vi "PGrafica.vi"() -> ()   [LabVIEW 2020]
uses:
  Pos_modifi.vi
  Llenado.vi
  sensores.vi
  Pos_iniciales.vi
  Pos_iniciales3.vi
  Pos_iniciales1.vi
panel:
  out "Piston C":bool
  out "Piston Abierto Y":i32
  out "Piston Abierto X":i32
  out "Sensor 1 Y":i32
  out "Laminadora":bool
  out "Caja Y":i32
  out "Caja X":i32
  out "Caja":bool
  out "Bote Pintado Y":i32
  out "Bote Pintado X":i32
  out "Bote cerrado Y":i32
  out "Bote cerrado X":i32
  out "Carrito Y":i32
  out "Carrito X":i32
  out "Pintura Y":i32
  out "Pintura X":i32
  out "Pintado":dbl(knob) scale=0.0..10.0
  out "Laminadora Y":i32
  out "Laminadora X":i32
  out "Piston cerrado Y":i32
  out "Piston cerrado X":i32
  out "Sensor 1":bool
  out "Bote":u8(slide) scale=0.0..100.0
  out "Mezc Y":i32
  out "Mezc X":i32
  out "Bote Y":i32
  out "Bote X":i32
  out "Sensor1 X":i32
  out "Llenador Y":i32
  out "Llenador X":i32
  out "Llenar":u8(slide) scale=0.0..100.0
  out "Tanque":u8(slide) scale=0.0..100.0
  out "Mezclador":dbl(slide) scale=0.0..10.0
  out "Carrito":bool
  out "Bote Cerrado":bool
  out "Bote Pintado":bool
  out "Piston A":bool
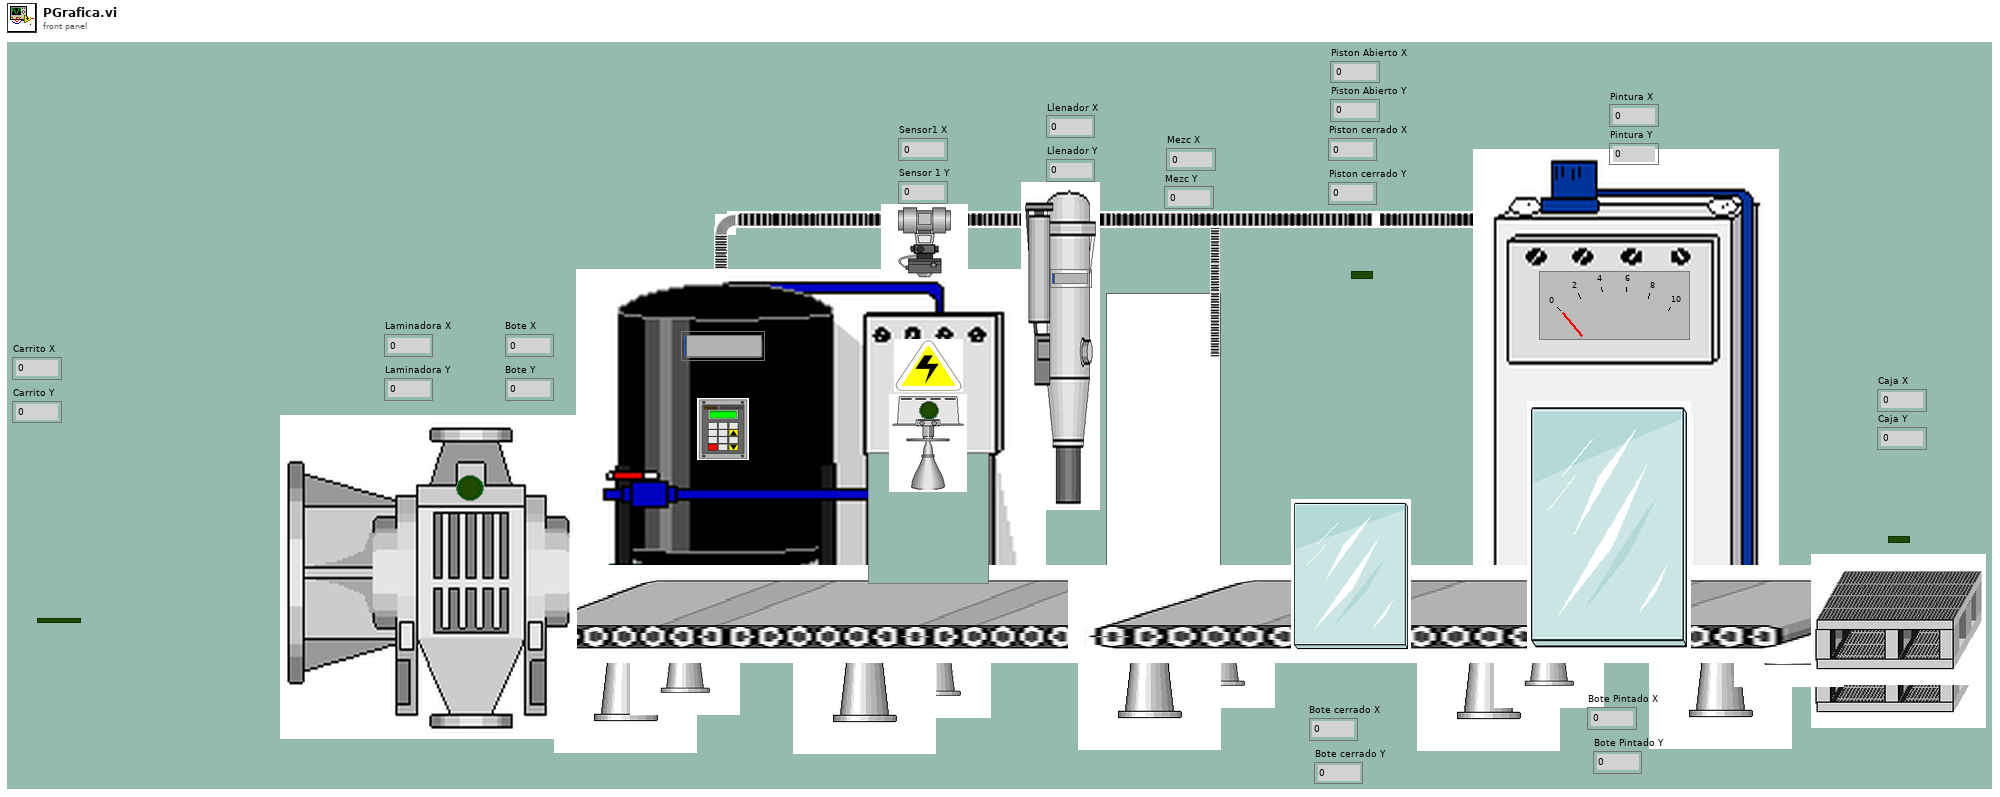
[diagram p1: front panel]
types:
  T1 = cluster{"Sensor 1":bool, "Laminadora":bool, "PistonA":bool, "PistonC":bool}
  T2 = cluster{"Bote":u8, "Llenador":u8, "Tanque":u8, "Pintado":dbl, "Mezclador":dbl}
  T3 = cluster{"Pos_Car":dbl, "Pos_lataAb":dbl, "Pos_lataCd":dbl, "Pos_lataPtd":dbl}
  T4 = cluster{"Pos_lataCX":dbl, "Pos_lataCY":dbl, "Pos_lataPX":dbl, "Pos_lataPY":dbl, "Pos_pintadoX":dbl, "Pos_pintadoY":dbl, "CajaX":dbl, "CajaY":dbl}
  T5 = cluster{"Pos_CarX":dbl, "Pos_Cary":dbl, "Pos_LamX":dbl, "Pos_LamY":dbl, "Pos_lataAX":dbl, "Pos_lataAy":dbl}
  T6 = cluster{"Pos_Snr1X":dbl, "Pos_SnrY":dbl, "Pos_LldrX":dbl, "Pos_LldrY":dbl, "Pos_MzdX":dbl, "Pos_MzdY":dbl, "Pos_PisX":dbl, "Pos_PisY":dbl}
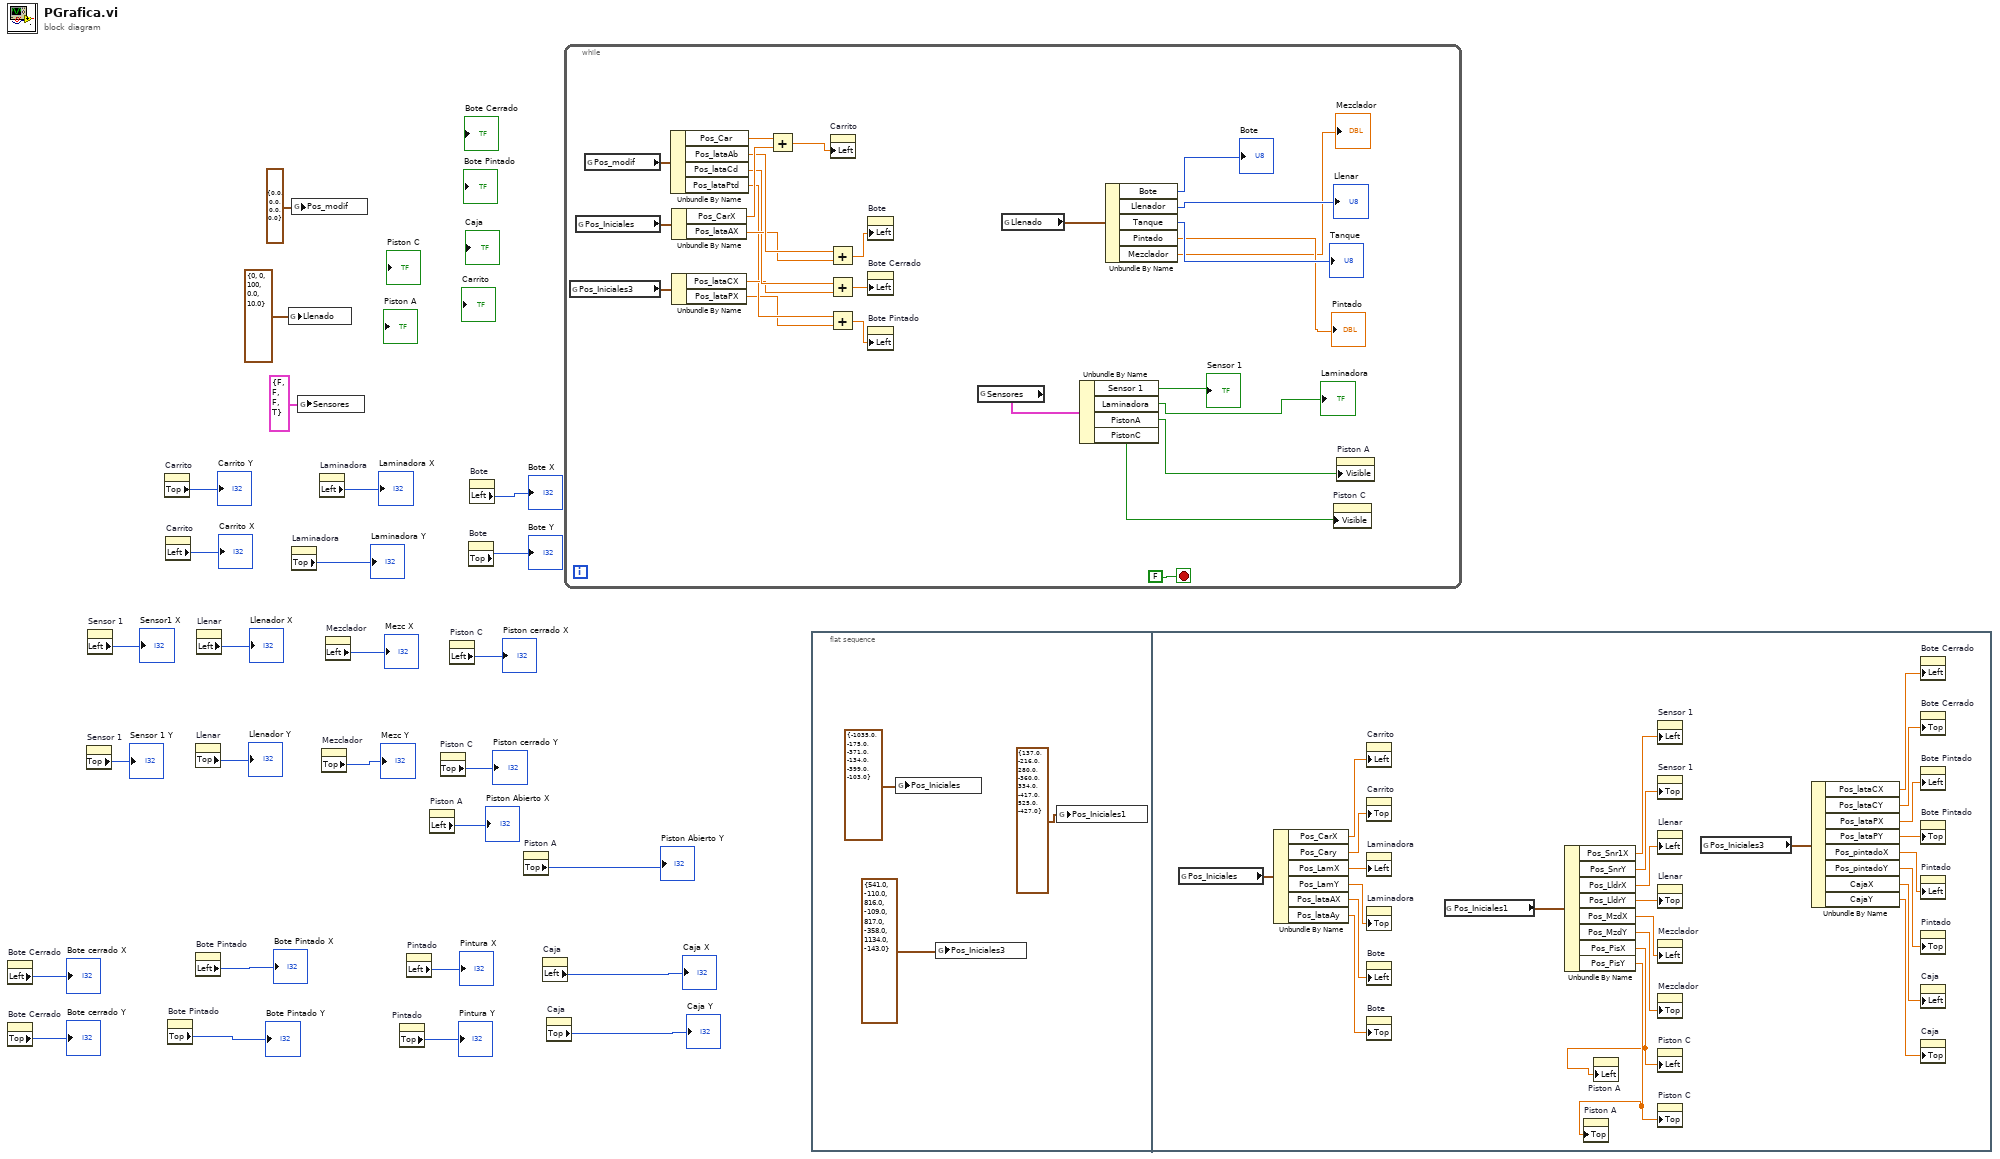
[diagram p0: block diagram]
diagram:
  n1 = property on="Bote Cerrado" class="Bool (strict)"() -> ("Left"=→"Bote cerrado X":i32)  [unwired: 2 in, 2 out]
  n2 = property on="Bote Cerrado" class="Bool (strict)"() -> ("Top"=→"Bote cerrado Y":i32)  [unwired: 2 in, 2 out]
  n3 = property on="Sensor 1" class="Bool (strict)"() -> ("Top"=→"Sensor 1 Y":i32)  [unwired: 2 in, 2 out]
  n4 = property on="Sensor 1" class="Bool (strict)"() -> ("Left"=→"Sensor1 X":i32)  [unwired: 2 in, 2 out]
  n5 = property on="Carrito" class="Bool (strict)"() -> ("Top"=→"Carrito Y":i32)  [unwired: 2 in, 2 out]
  n6 = property on="Carrito" class="Bool (strict)"() -> ("Left"=→"Carrito X":i32)  [unwired: 2 in, 2 out]
  n7 = property on="Bote Pintado" class="Bool (strict)"() -> ("Top"=→"Bote Pintado Y":i32)  [unwired: 2 in, 2 out]
  n8 = property on="Llenar" class="Slide (strict)"() -> ("Top"=→"Llenador Y":i32)  [unwired: 2 in, 2 out]
  n9 = property on="Bote Pintado" class="Bool (strict)"() -> ("Left"=→"Bote Pintado X":i32)  [unwired: 2 in, 2 out]
  n10 = property on="Llenar" class="Slide (strict)"() -> ("Left"=→"Llenador X":i32)  [unwired: 2 in, 2 out]
  n11 = global write "Llenado.vi" "Llenado"(T2 {"Bote"=0, "Llenador"=0, "Tanque"=100, "Pintado"=0.0, "Mezclador"=10.0} ("Llenado")) -> ()
  n12 = global write "Pos_modifi.vi" "Pos_modif"(T3 {"Pos_Car"=0.0, "Pos_lataAb"=0.0, "Pos_lataCd"=0.0, "Pos_lataPtd"=0.0} ("Pos_modif")) -> ()
  n13 = property on="Laminadora" class="Bool (strict)"() -> ("Top"=→"Laminadora Y":i32)  [unwired: 2 in, 2 out]
  n14 = global write "sensores.vi" "Sensores"(T1 {"Sensor 1"=FALSE, "Laminadora"=FALSE, "PistonA"=FALSE, "PistonC"=TRUE} ("Sensores")) -> ()
  n15 = property on="Laminadora" class="Bool (strict)"() -> ("Left"=→"Laminadora X":i32)  [unwired: 2 in, 2 out]
  n16 = property on="Mezclador" class="Slide (strict)"() -> ("Top"=→"Mezc Y":i32)  [unwired: 2 in, 2 out]
  n17 = property on="Mezclador" class="Slide (strict)"() -> ("Left"=→"Mezc X":i32)  [unwired: 2 in, 2 out]
  n18 = property on="Pintado" class="Knob (strict)"() -> ("Top"=→"Pintura Y":i32)  [unwired: 2 in, 2 out]
  n19 = property on="Pintado" class="Knob (strict)"() -> ("Left"=→"Pintura X":i32)  [unwired: 2 in, 2 out]
  n20 = property on="Piston A" class="Bool (strict)"() -> ("Left"=→"Piston Abierto X":i32)  [unwired: 2 in, 2 out]
  n21 = property on="Piston C" class="Bool (strict)"() -> ("Top"=→"Piston cerrado Y":i32)  [unwired: 2 in, 2 out]
  n22 = property on="Piston C" class="Bool (strict)"() -> ("Left"=→"Piston cerrado X":i32)  [unwired: 2 in, 2 out]
  n23 = property on="Bote" class="Slide (strict)"() -> ("Top"=→"Bote Y":i32)  [unwired: 2 in, 2 out]
  n24 = property on="Bote" class="Slide (strict)"() -> ("Left"=→"Bote X":i32)  [unwired: 2 in, 2 out]
  n25 = property on="Piston A" class="Bool (strict)"() -> ("Top"=→"Piston Abierto Y":i32)  [unwired: 2 in, 2 out]
  n26 = property on="Caja" class="Bool (strict)"() -> ("Left"=→"Caja X":i32)  [unwired: 2 in, 2 out]
  n27 = property on="Caja" class="Bool (strict)"() -> ("Top"=→"Caja Y":i32)  [unwired: 2 in, 2 out]
  n28 = while {
    stop <- FALSE stop-if-true
    n29 = global read "Pos_iniciales3.vi" "Pos_Iniciales3"() -> (w51:T4)
    n30 = global read "Pos_iniciales.vi" "Pos_Iniciales"() -> (w52:T5)
    n31 = global read "Pos_modifi.vi" "Pos_modif"() -> (w53:T3)
    n32 = Unbundle By Name(w53) -> ("Pos_Car"=w50:dbl, "Pos_lataAb"=w48:dbl, "Pos_lataCd"=w46:dbl, "Pos_lataPtd"=w44:dbl)
    n33 = Unbundle By Name(w52) -> ("Pos_CarX"=w49:dbl, "Pos_lataAX"=w47:dbl)
    n34 = Unbundle By Name(w51) -> ("Pos_lataCX"=w45:dbl, "Pos_lataPX"=w43:dbl)
    n35 = Add(x=w50, y=w49) -> (x+y=w39:dbl)
    n36 = Add(x=w48, y=w47) -> (x+y=w42:dbl)
    n37 = Add(x=w46, y=w45) -> (x+y=w41:dbl)
    n38 = Add(x=w44, y=w43) -> (x+y=w40:dbl)
    n39 = property on="Carrito" class="Bool (strict)"("Left"=w39) -> ()  [unwired: 2 in, 2 out]
    n40 = property on="Bote" class="Slide (strict)"("Left"=w42) -> ()  [unwired: 2 in, 2 out]
    n41 = property on="Bote Cerrado" class="Bool (strict)"("Left"=w41) -> ()  [unwired: 2 in, 2 out]
    n42 = property on="Bote Pintado" class="Bool (strict)"("Left"=w40) -> ()  [unwired: 2 in, 2 out]
    n43 = global read "sensores.vi" "Sensores"() -> (w32:T1)
    n44 = global read "Llenado.vi" "Llenado"() -> (w38:T2)
    n45 = Unbundle By Name(w32) -> ("Sensor 1"=→"Sensor 1":bool, "Laminadora"=→"Laminadora":bool, "PistonA"=w29:bool, "PistonC"=w28:bool)
    n46 = Unbundle By Name(w38) -> ("Bote"=→"Bote":u8, "Llenador"=→"Llenar":u8, "Tanque"=→"Tanque":u8, "Pintado"=→"Pintado":dbl, "Mezclador"=→"Mezclador":dbl)
    n47 = property on="Piston C" class="Bool (strict)"("Visible"=w28) -> ()  [unwired: 2 in, 2 out]
    n48 = property on="Piston A" class="Bool (strict)"("Visible"=w29) -> ()  [unwired: 2 in, 2 out]
  }
  n49 = flat-sequence {
    frame #0 {
      n50 = global write "Pos_iniciales.vi" "Pos_Iniciales"(T5 {"Pos_CarX"=-1035.0, "Pos_Cary"=-175.0, "Pos_LamX"=-371.0, "Pos_LamY"=-134.0, "Pos_lataAX"=-399.0, "Pos_lataAy"=-103.0} ("Pos_Iniciales")) -> ()
      n51 = global write "Pos_iniciales3.vi" "Pos_Iniciales3"(T4 {"Pos_lataCX"=541.0, "Pos_lataCY"=-110.0, "Pos_lataPX"=816.0, "Pos_lataPY"=-109.0, "Pos_pintadoX"=817.0, "Pos_pintadoY"=-358.0, "CajaX"=1134.0, "CajaY"=-143.0} ("Cluster")) -> ()
      n52 = global write "Pos_iniciales1.vi" "Pos_Iniciales1"(T6 {"Pos_Snr1X"=137.0, "Pos_SnrY"=-216.0, "Pos_LldrX"=280.0, "Pos_LldrY"=-360.0, "Pos_MzdX"=334.0, "Pos_MzdY"=-417.0, "Pos_PisX"=525.0, "Pos_PisY"=-427.0} ("Cluster")) -> ()
    }
    frame #1 {
      n53 = global read "Pos_iniciales.vi" "Pos_Iniciales"() -> (w76:T5)
      n54 = Unbundle By Name(w76) -> ("Pos_CarX"=w77:dbl, "Pos_Cary"=w78:dbl, "Pos_LamX"=w79:dbl, "Pos_LamY"=w80:dbl, "Pos_lataAX"=w81:dbl, "Pos_lataAy"=w82:dbl)
      n55 = property on="Carrito" class="Bool (strict)"("Left"=w77) -> ()  [unwired: 2 in, 2 out]
      n56 = property on="Carrito" class="Bool (strict)"("Top"=w78) -> ()  [unwired: 2 in, 2 out]
      n57 = property on="Laminadora" class="Bool (strict)"("Left"=w79) -> ()  [unwired: 2 in, 2 out]
      n58 = property on="Laminadora" class="Bool (strict)"("Top"=w80) -> ()  [unwired: 2 in, 2 out]
      n59 = property on="Bote" class="Slide (strict)"("Left"=w81) -> ()  [unwired: 2 in, 2 out]
      n60 = property on="Bote" class="Slide (strict)"("Top"=w82) -> ()  [unwired: 2 in, 2 out]
      n61 = global read "Pos_iniciales1.vi" "Pos_Iniciales1"() -> (w67:T6)
      n62 = Unbundle By Name(w67) -> ("Pos_Snr1X"=w68:dbl, "Pos_SnrY"=w69:dbl, "Pos_LldrX"=w70:dbl, "Pos_LldrY"=w71:dbl, "Pos_MzdX"=w72:dbl, "Pos_MzdY"=w73:dbl, "Pos_PisX"=w74:dbl, "Pos_PisY"=w75:dbl)
      n63 = property on="Piston A" class="Bool (strict)"("Top"=w75) -> ()  [unwired: 2 in, 2 out]
      n64 = property on="Piston A" class="Bool (strict)"("Left"=w74) -> ()  [unwired: 2 in, 2 out]
      n65 = property on="Sensor 1" class="Bool (strict)"("Left"=w68) -> ()  [unwired: 2 in, 2 out]
      n66 = property on="Sensor 1" class="Bool (strict)"("Top"=w69) -> ()  [unwired: 2 in, 2 out]
      n67 = property on="Llenar" class="Slide (strict)"("Left"=w70) -> ()  [unwired: 2 in, 2 out]
      n68 = property on="Llenar" class="Slide (strict)"("Top"=w71) -> ()  [unwired: 2 in, 2 out]
      n69 = property on="Mezclador" class="Slide (strict)"("Left"=w72) -> ()  [unwired: 2 in, 2 out]
      n70 = property on="Mezclador" class="Slide (strict)"("Top"=w73) -> ()  [unwired: 2 in, 2 out]
      n71 = property on="Piston C" class="Bool (strict)"("Left"=w74) -> ()  [unwired: 2 in, 2 out]
      n72 = property on="Piston C" class="Bool (strict)"("Top"=w75) -> ()  [unwired: 2 in, 2 out]
      n73 = global read "Pos_iniciales3.vi" "Pos_Iniciales3"() -> (w58:T4)
      n74 = Unbundle By Name(w58) -> ("Pos_lataCX"=w59:dbl, "Pos_lataCY"=w60:dbl, "Pos_lataPX"=w61:dbl, "Pos_lataPY"=w62:dbl, "Pos_pintadoX"=w63:dbl, "Pos_pintadoY"=w64:dbl, "CajaX"=w65:dbl, "CajaY"=w66:dbl)
      n75 = property on="Bote Cerrado" class="Bool (strict)"("Left"=w59) -> ()  [unwired: 2 in, 2 out]
      n76 = property on="Bote Cerrado" class="Bool (strict)"("Top"=w60) -> ()  [unwired: 2 in, 2 out]
      n77 = property on="Bote Pintado" class="Bool (strict)"("Left"=w61) -> ()  [unwired: 2 in, 2 out]
      n78 = property on="Bote Pintado" class="Bool (strict)"("Top"=w62) -> ()  [unwired: 2 in, 2 out]
      n79 = property on="Pintado" class="Knob (strict)"("Left"=w63) -> ()  [unwired: 2 in, 2 out]
      n80 = property on="Pintado" class="Knob (strict)"("Top"=w64) -> ()  [unwired: 2 in, 2 out]
      n81 = property on="Caja" class="Bool (strict)"("Left"=w65) -> ()  [unwired: 2 in, 2 out]
      n82 = property on="Caja" class="Bool (strict)"("Top"=w66) -> ()  [unwired: 2 in, 2 out]
    }
  }
